vi "Get logged in user.vi"(11 "Refnum in":T3) -> (2 "User Logged in":bool, 3 "user login":T1)   [LabVIEW 2024, in "DB.lvlib"]
uses:
  DB.lvlib
  <vilib>/addons/database/Connection.llb/Conn ObjectReference.ctl
  Controls/Login info.ctl
  Controls/User level.ctl
  <vilib>/addons/database/NI_Database_API.lvlib
panel:
  out "error out":errorcluster
  in  "error in (no error)":errorcluster
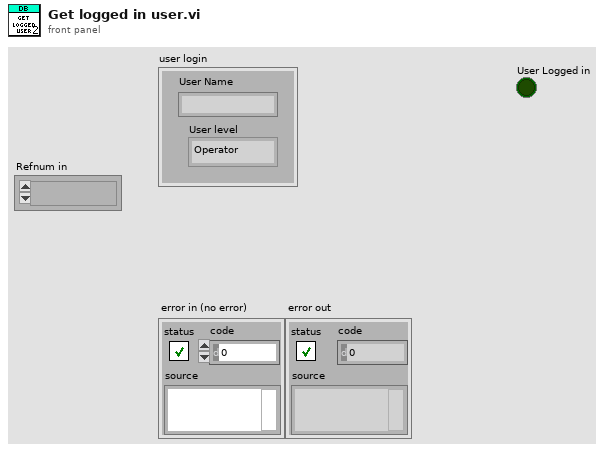
[diagram p1: front panel]
types:
  T1 = typedef "Login info.ctl" = cluster{"User Name":string, "User level":T2}
  T2 = typedef "User level.ctl" = enum16{"Operator", "Admin"}
  T3 = typedef "NI_Database_API.lvlib/Conn ObjectReference.ctl" = refnum<k1>
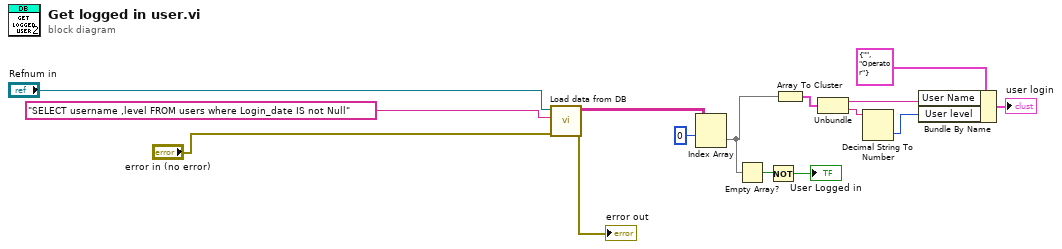
[diagram p0: block diagram]
diagram:
  n1 = call "Load data from DB.vi"("error in (no error)"="error in (no error)", "SQL query"="SELECT username ,level FROM users where Login_date IS not Null", "Refnum in"="Refnum in") -> ("error out"=→"error out":errorcluster, "Array"=w15:string[][])  [unwired: 7 in]
  n2 = Index Array(array=w15, index (row)=0) -> (element=w8:string[])  [unwired: 1 in]
  n3 = Empty Array?(array=w8) -> (empty?=w10:bool)
  n4 = Not(x=w10) -> (.not. x?=→"User Logged in":bool)
  n5 = Array To Cluster(array=w8) -> (cluster=w7:cluster{"Array[0]":string, "Array[1]":string})
  n6 = Unbundle(w7) -> ("Array[0]"=w5:string, "Array[1]"=w3:string)
  n7 = Decimal String To Number(string=w3) -> (number=w2:i32)  [unwired: 2 in, 1 out]
  n8 = Bundle By Name(cluster=T1 {"User Name"="", "User level"=enum."Operator"} ("Login info"), "User Name"=w5, "User level"=w2) -> (→"user login":T1)
